vi "多帧接收机制(EV05).vi"(0 "can卡类型":u8, 1 "设备索引号":u8, 2 "CAN端口":u8, 3 "VCI_Receive":T1 {"Rsv3" max=0 format="%x"; "Rsv2" min=101 format="%x"; "Rsv1" format="%x"; "Data8" format="%x"; "Data7" format="%x"; "Data6" format="%x"; "Data5" format="%x"; "Data4" format="%x"; "Data3" format="%x"; "Data2" format="%x"; "Data1" format="%x"; "DataLen" format="%x"; "ExternFlag" format="%x"; "RemoteFlag" format="%x"; "SendType" format="%x"; "TimeFlag" format="%x"; "TimeStamp" format="%x"; "ID" format="%x"}, 4 "命令":u32 format="%x", 5 "板号":u32 format="%x", 7 "写?":bool, 9 "命令序号":u8) -> (13 "错误信号":bool, 14 "错误代码":i32, 15 "多帧数据长度":i32, 16 "命令序号":u8, 17 "输出数组":u8[](array[numeric]), 18 "读错误代码":u8[](array[numeric]), 19 "结束信号":bool)   [LabVIEW 2013]
panel:
  in  "最大帧号":i32
  out "多帧个数":i32
  out "长度1":i32
  out "接收完成":bool
  in  "多帧计时":bool
  in  "Reset 2":bool caption="重置"
  in  "Reset":bool caption="重置"
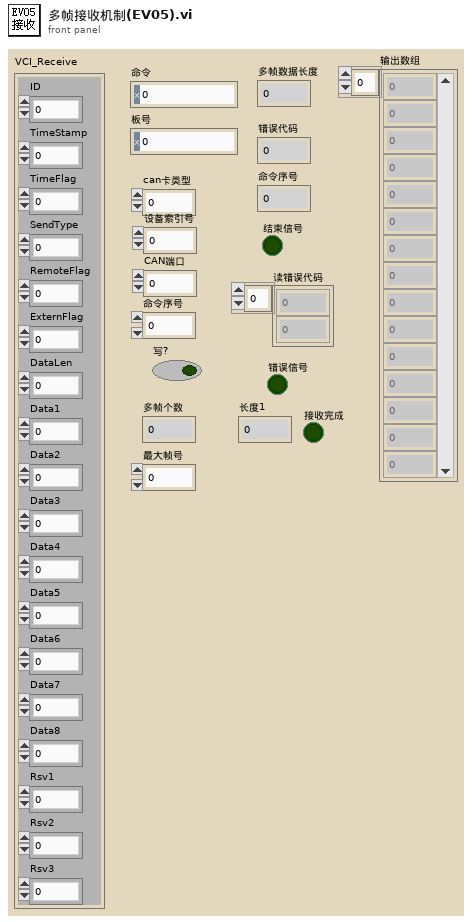
[diagram p1: front panel]
types:
  T1 = cluster{"ID":u32, "TimeStamp":u32, "TimeFlag":u8, "SendType":u8, "RemoteFlag":u8, "ExternFlag":u8, "DataLen":u8, "Data1":u8, "Data2":u8, "Data3":u8, "Data4":u8, "Data5":u8, "Data6":u8, "Data7":u8, "Data8":u8, "Rsv1":u8, "Rsv2":u8, "Rsv3":u8}
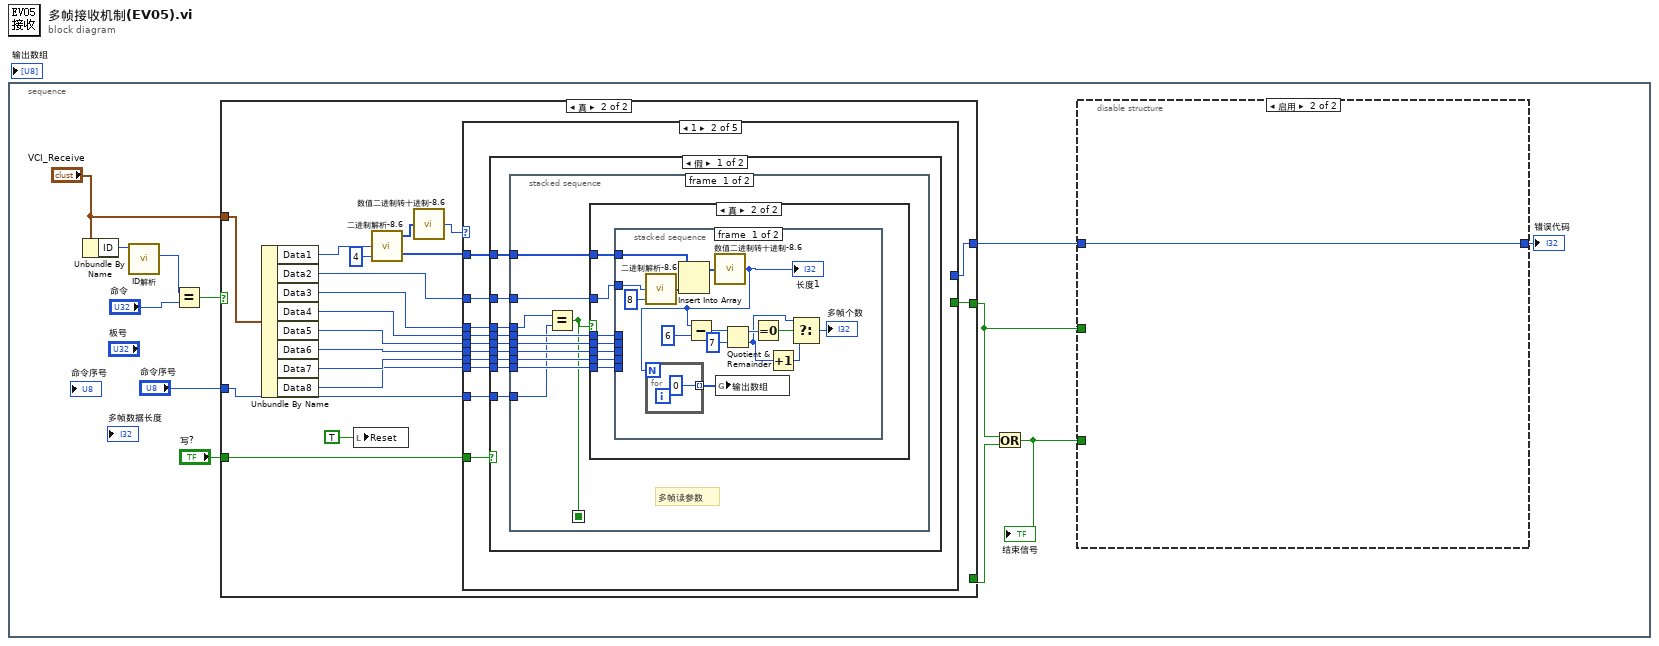
[diagram p0: block diagram]
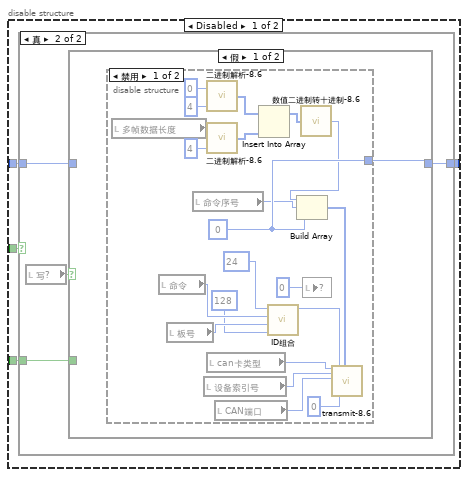
[diagram p2: hidden frame]
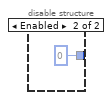
[diagram p4: hidden frame]
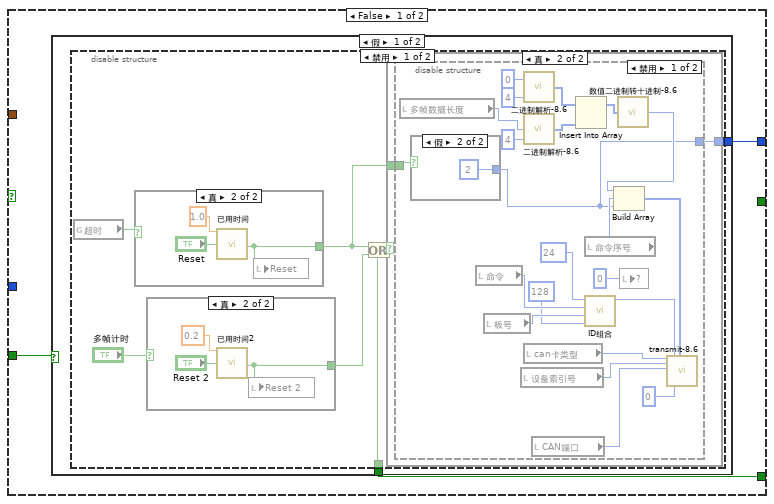
[diagram p6: hidden frame]
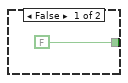
[diagram p8: hidden frame]
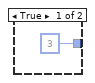
[diagram p10: hidden frame]
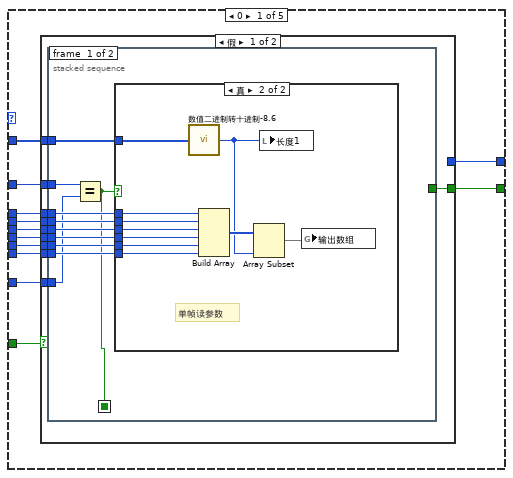
[diagram p14: hidden frame]
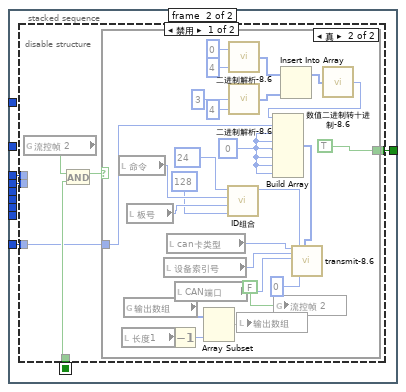
[diagram p16: hidden frame]
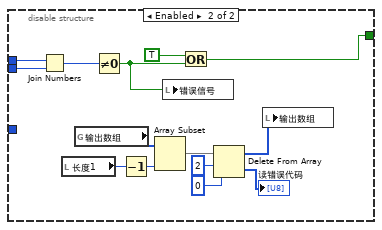
[diagram p18: hidden frame]
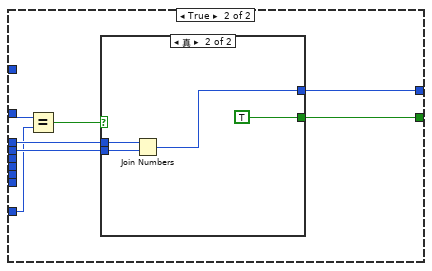
[diagram p19: hidden frame]
diagram:
  n1 = stacked-sequence {
    frame #0 {
      n2 = Unbundle By Name("VCI_Receive") -> ("ID"=w12:u32)
      n3 = call "ID解析.vi"("ID"=w12) -> ("PF(2)"=w11:i32)  [unwired: 10 out]
      n4 = Equal?(x=w11, y="命令") -> (x = y?=w5:bool)
      n5 = case shown="真" w5 {
        tunnel: "VCI_Receive" -> [_ w108]
        tunnel: [_ w94] -> w8
        tunnel: [w49 _] -> w4
        tunnel: [w48 w93] -> w7
        tunnel: "写?" -> [w47 w92]
        tunnel: "命令序号" -> [_ w91]
        frame False {
          n6 = case shown="假" w47 {
            tunnel: [w51 _] -> w49
            tunnel: [w50 _] -> w48
            frame False {
              n7 = disable-structure shown="禁用" {
                disable-tunnel: [w54 _] -> w51
                disable-tunnel: [w53 _] -> w50
                frame Disabled {
                  n8 = global read "EV05全局变量1.vi" "超时"() -> (w52:bool)
                  n9 = case shown="真" w52 {
                    tunnel: [_ w60] -> w56
                    frame False {
                    }
                    frame True {
                      n10 = call "已用时间"("Time Target (s)"=1.0, "Reset"="Reset") -> ("Time has Elapsed"=w60:bool)  [unwired: 3 in, 14 out]
                      n11 = local write "Reset"(w60) -> ()
                    }
                  }
                  n12 = case shown="真" "多帧计时" {
                    tunnel: [FALSE ("Time has Elapsed") w62] -> w55
                    frame False {
                    }
                    frame True {
                      n13 = call "已用时间2"("Time Target (s)"=0.2, "Reset"="Reset 2") -> ("Time has Elapsed"=w62:bool)  [unwired: 3 in, 14 out]
                      n14 = local write "Reset 2"(w62) -> ()
                    }
                  }
                  n15 = Or(x=w56, y=w55) -> (x .or. y?=w54:bool)
                  n16 = case shown="真" w54 {
                    tunnel: w56 -> [_ w66]
                    tunnel: [_ w65] -> w53
                    frame False {
                    }
                    frame True {
                      n17 = disable-structure shown="禁用" {
                        disable-tunnel: w66 -> [w81 _]
                        disable-tunnel: [w70 _] -> w65
                        frame Disabled {
                          n18 = local read "多帧数据长度"() -> (w72:i32)
                          n19 = case shown="假" w81 {
                            tunnel: [3 ("元素") 2 ("元素")] -> w70
                            frame True {
                            }
                            frame False {
                            }
                          }
                          n20 = local read "命令"() -> (w84:u32)
                          n21 = local read "板号"() -> (w69:u32)
                          n22 = local read "设备索引号"() -> (w87:u8)
                          n23 = call "二进制解析-8.6.vi"("索引"=4, "数值"=0) -> ("低位子数组"=w75:i32[])  [unwired: 3 out]
                          n24 = call "二进制解析-8.6.vi"("索引"=4, "数值"=w72) -> ("低位子数组"=w74:i32[])  [unwired: 3 out]
                          n25 = local read "can卡类型"() -> (w88:u8)
                          n26 = local read "CAN端口"() -> (w86:u8)
                          n27 = Insert Into Array(array=w75, new element=w74) -> (w73:i32[])  [unwired: 1 in]
                          n28 = local read "命令序号"() -> (w80:u8)
                          n29 = call "ID组合.vi"("SA(4)"=128 ("PDU(1)"), "PS(3)"=w69, "PF(2)"=w84, "PDU(1)"=24) -> ("ID"=w83:i32)  [unwired: 7 out]
                          n30 = call "数值二进制转十进制-8.6.vi"("子数组"=w73) -> ("十进制数值"=w71:i32)  [unwired: 4 out]
                          n31 = Build Array(w71, w80, w70) -> (w82:i32[])
                          n32 = local write item#-1(u8 0 ("计数")) -> ()
                          n33 = call "transmit-8.6.vi"("can卡类型"=w88, "设备索引号"=w87, "CAN端口"=w86, "ID"=w83, "SendType"=u8 0, "Data"=w82) -> ()  [unwired: 3 in, 11 out]
                        }
                        frame Enabled {
                        }
                      }
                    }
                  }
                }
                frame Enabled {
                }
              }
            }
            frame True {
            }
          }
        }
        frame True {
          n34 = Unbundle By Name(w108) -> ("Data1"=w107:u8, "Data2"=w103:u8, "Data3"=w101:u8, "Data4"=w100:u8, "Data5"=w99:u8, "Data6"=w98:u8, "Data7"=w97:u8, "Data8"=w96:u8)
          n35 = local write "Reset"(TRUE ("Reset")) -> ()
          n36 = call "二进制解析-8.6.vi"("索引"=4, "数值"=w107) -> ("低位子数组"=w102:i32[], "高位子数组"=w105:i32[])  [unwired: 2 out]
          n37 = call "数值二进制转十进制-8.6.vi"("子数组"=w105) -> ("十进制数值"=w104:i32)  [unwired: 4 out]
          n38 = case shown="1" w104 {
            tunnel: w103 -> [w120 w221 w307 _ _]
            tunnel: w102 -> [w119 w220 w309 _ _]
            tunnel: w101 -> [w113 w219 w308 _ _]
            tunnel: w100 -> [w118 w218 w306 _ _]
            tunnel: w99 -> [w117 w217 w305 _ _]
            tunnel: w98 -> [w116 w216 w304 _ _]
            tunnel: w97 -> [w115 w215 w303 _ _]
            tunnel: w96 -> [w114 w214 w302 _ _]
            tunnel: [w110 _ w299 _ _] -> w94
            tunnel: [w112 _ _ _ _] -> w93
            tunnel: w92 -> [w111 w213 w298 _ _]
            tunnel: w91 -> [w109 w212 _ _ _]
            frame 0 {
              n39 = case shown="假" w111 {
                tunnel: w120 -> [w130 w203]
                tunnel: w119 -> [w129 _]
                tunnel: w118 -> [w128 w205]
                tunnel: w117 -> [w127 _]
                tunnel: w116 -> [w126 _]
                tunnel: w115 -> [w125 _]
                tunnel: w114 -> [w124 _]
                tunnel: w113 -> [w123 w206]
                tunnel: [_ w207] -> w112
                tunnel: [w122 w204] -> w110
                tunnel: w109 -> [w121 w202]
                frame False {
                  n40 = stacked-sequence {
                    seq-local: [w131 _] -> [_ w154]
                    tunnel: w130 -> [w133 _]
                    tunnel: w129 -> [w140 _]
                    tunnel: w128 -> [w139 w151]
                    tunnel: w127 -> [w138 _]
                    tunnel: w126 -> [w137 _]
                    tunnel: w125 -> [w136 _]
                    tunnel: w124 -> [w135 _]
                    tunnel: w123 -> [w134 w152]
                    tunnel: [_ w155] -> w122
                    tunnel: w121 -> [w132 w153]
                    frame #0 {
                      n41 = Equal?(x=w133, y=w132) -> (x = y?=w131:bool)
                      n42 = case shown="真" w131 {
                        tunnel: w140 -> [_ w150]
                        tunnel: w139 -> [_ w149]
                        tunnel: w138 -> [_ w148]
                        tunnel: w137 -> [_ w147]
                        tunnel: w136 -> [_ w146]
                        tunnel: w135 -> [_ w145]
                        tunnel: w134 -> [_ w144]
                        frame False {
                        }
                        frame True {
                          # "单帧读参数"
                          n43 = call "数值二进制转十进制-8.6.vi"("子数组"=w150) -> ("十进制数值"=w142:i32)  [unwired: 4 out]
                          n44 = Build Array(w144, w149, w148, w147, w146, w145) -> (w143:u8[])
                          n45 = Array Subset(array=w143, length=w142) -> (w141:u8[])  [unwired: 1 in]
                          n46 = local write "长度1"(w142) -> ()
                          n47 = global write "EV05全局变量1.vi" "输出数组"(w141) -> ()
                        }
                      }
                    }
                    frame #1 {
                      n48 = disable-structure shown="禁用" {
                        disable-tunnel: [w160 w189] -> w155
                        disable-tunnel: w154 -> [w159 _]
                        disable-tunnel: w153 -> [w156 _]
                        disable-tunnel: w152 -> [_ w195]
                        disable-tunnel: w151 -> [_ w196]
                        frame Disabled {
                          n49 = global read "EV05全局变量1.vi" "流控帧 2"() -> (w157:bool)
                          n50 = And(x=w157, y=w159) -> (x .and. y?=w158:bool)
                          n51 = case shown="真" w158 {
                            tunnel: [_ TRUE] -> w160
                            tunnel: w156 -> [_ w163]
                            frame False {
                            }
                            frame True {
                              w179 = 0 ("元素")
                              n52 = local read "命令"() -> (w182:u32)
                              n53 = local read "长度1"() -> (w165:i32)
                              n54 = global read "EV05全局变量1.vi" "输出数组"() -> (w167:u8[])
                              n55 = local read "板号"() -> (w171:u32)
                              n56 = local read "设备索引号"() -> (w185:u8)
                              n57 = local read "can卡类型"() -> (w186:u8)
                              n58 = Decrement(x=w165) -> (x-1=w164:i32)
                              n59 = local read "CAN端口"() -> (w184:u8)
                              n60 = Array Subset(array=w167, length=w164) -> (w166:u8[])  [unwired: 1 in]
                              n61 = call "ID组合.vi"("SA(4)"=128 ("PDU(1)"), "PS(3)"=w171, "PF(2)"=w182, "PDU(1)"=24) -> ("ID"=w181:i32)  [unwired: 7 out]
                              n62 = call "二进制解析-8.6.vi"("索引"=4, "数值"=0) -> ("低位子数组"=w175:i32[])  [unwired: 3 out]
                              n63 = call "二进制解析-8.6.vi"("索引"=4, "数值"=3) -> ("低位子数组"=w172:i32[])  [unwired: 3 out]
                              n64 = local write "输出数组"(w166) -> ()
                              n65 = global write "EV05全局变量1.vi" "流控帧 2"(FALSE ("流控帧 2")) -> ()
                              n66 = Insert Into Array(array=w175, new element=w172) -> (w174:i32[])  [unwired: 1 in]
                              n67 = call "数值二进制转十进制-8.6.vi"("子数组"=w174) -> ("十进制数值"=w173:i32)  [unwired: 4 out]
                              n68 = Build Array(w173, w163, w179, w179, w179, w179, w179, w179) -> (w180:i32[])
                              n69 = call "transmit-8.6.vi"("can卡类型"=w186, "设备索引号"=w185, "CAN端口"=w184, "ID"=w181, "SendType"=u8 0, "Data"=w180) -> ()  [unwired: 3 in, 11 out]
                            }
                          }
                        }
                        frame Enabled {
                          n70 = Join Numbers(hi=w195, lo=w196) -> ((hi.lo)=w194:u16)
                          n71 = local read "长度1"() -> (w198:i32)
                          n72 = global read "EV05全局变量1.vi" "输出数组"() -> (w200:u8[])
                          n73 = Not Equal To 0?(x=w194) -> (x != 0?=w187:bool)
                          n74 = Decrement(x=w198) -> (x-1=w197:i32)
                          n75 = Array Subset(array=w200, length=w197) -> (w199:u8[])  [unwired: 1 in]
                          n76 = local write "错误信号"(w187) -> ()
                          n77 = Or(x=TRUE, y=w187) -> (x .or. y?=w189:bool)
                          n78 = Delete From Array(array=w199, length=2 ("长度"), index=0 ("索引")) -> (deleted portion=→"读错误代码":u8[], array with subset deleted=w193:u8[])
                          n79 = local write "输出数组"(w193) -> ()
                        }
                      }
                    }
                  }
                }
                frame True {
                  n80 = Equal?(x=w203, y=w202) -> (x = y?=w201:bool)
                  n81 = case shown="真" w201 {
                    tunnel: [_ w211] -> w207
                    tunnel: w206 -> [_ w210]
                    tunnel: w205 -> [_ w209]
                    tunnel: [_ TRUE] -> w204
                    frame False {
                    }
                    frame True {
                      n82 = Join Numbers(hi=w210, lo=w209) -> ((hi.lo)=w211:u16)
                    }
                  }
                }
              }
            }
            frame 1 {
              n83 = case shown="假" w213 {
                tunnel: w221 -> [w230 _]
                tunnel: w220 -> [w229 _]
                tunnel: w219 -> [w228 _]
                tunnel: w218 -> [w227 _]
                tunnel: w217 -> [w226 _]
                tunnel: w216 -> [w225 _]
                tunnel: w215 -> [w224 _]
                tunnel: w214 -> [w223 _]
                tunnel: w212 -> [w222 _]
                frame False {
                  n84 = stacked-sequence {
                    seq-local: [w231 _] -> [_ w276]
                    tunnel: w230 -> [w240 _]
                    tunnel: w229 -> [w239 _]
                    tunnel: w228 -> [w233 _]
                    tunnel: w227 -> [w238 _]
                    tunnel: w226 -> [w237 _]
                    tunnel: w225 -> [w236 _]
                    tunnel: w224 -> [w235 _]
                    tunnel: w223 -> [w234 _]
                    tunnel: w222 -> [w232 _]
                    frame #0 {
                      # "多帧读参数"
                      n85 = Equal?(x=w233, y=w232) -> (x = y?=w231:bool)
                      n86 = case shown="真" w231 {
                        tunnel: w240 -> [_ w247]
                        tunnel: w239 -> [_ w246]
                        tunnel: w238 -> [_ w245]
                        tunnel: w237 -> [_ w244]
                        tunnel: w236 -> [_ w243]
                        tunnel: w235 -> [_ w242]
                        tunnel: w234 -> [_ w241]
                        frame False {
                        }
                        frame True {
                          n87 = stacked-sequence {
                            tunnel: w247 -> [w261 _]
                            tunnel: w246 -> [w259 _]
                            tunnel: w245 -> [_ w273]
                            tunnel: w244 -> [_ w272]
                            tunnel: w243 -> [_ w271]
                            tunnel: w242 -> [_ w270]
                            tunnel: w241 -> [_ w269]
                            frame #0 {
                              n88 = call "二进制解析-8.6.vi"("索引"=8, "数值"=w261) -> ("低位子数组"=w260:i32[])  [unwired: 3 out]
                              n89 = Insert Into Array(array=w259, new element=w260) -> (w258:i32[])  [unwired: 1 in]
                              n90 = call "数值二进制转十进制-8.6.vi"("子数组"=w258) -> ("十进制数值"=w256:i32)  [unwired: 4 out]
                              "长度1" <- w256
                              n91 = for {
                                N: w256 -> [_]
                                tunnel: [u8 0] -> w257 mode=indexing
                              }
                              n92 = Subtract(x=w256, y=6) -> (x-y=w254:i32)
                              n93 = global write "EV05全局变量1.vi" "输出数组"(w257) -> ()
                              n94 = Quotient & Remainder(x=w254, y=7) -> (x-y*floor(x/y)=w252:i32, floor(x/y)=w250:i32)
                              n95 = Equal To 0?(x=w252) -> (x = 0?=w251:bool)
                              n96 = Increment(x=w250) -> (x+1=w249:i32)
                              n97 = Select(t=w250, s=w251, f=w249) -> (s? t:f=→"多帧个数":i32)
                            }
                            frame #1 {
                              # "收第一帧5字节数据"
                              n98 = Build Array(w273, w272, w271, w270, w269) -> (w267:u8[])
                              n99 = global read "EV05全局变量1.vi" "输出数组"() -> (w268:u8[])
                              n100 = local write "最大帧号"(1 ("最大帧号")) -> ()
                              n101 = Replace Array Subset(array=w268, new element=w267, index=0 ("索引")) -> (w266:u8[])
                              n102 = global write "EV05全局变量1.vi" "输出数组"(w266) -> ()
                            }
                          }
                        }
                      }
                    }
                    frame #1 {
                      n103 = global read "EV05全局变量1.vi" "流控帧 2"() -> (w274:bool)
                      n104 = And(x=w274, y=w276) -> (x .and. y?=w275:bool)
                      n105 = case shown="真" w275 {
                        frame False {
                        }
                        frame True {
                          w283 = 0 ("元素")
                          n106 = local read "命令"() -> (w284:u32)
                          n107 = local read "板号"() -> (w280:u32)
                          n108 = call "ID组合.vi"("SA(4)"=145 ("PDU(1)"), "PS(3)"=w280, "PF(2)"=w284, "PDU(1)"=24) -> ("ID"=w286:i32)  [unwired: 7 out]
                          n109 = call "二进制解析-8.6.vi"("索引"=4, "数值"=3) -> ("低位子数组"=w291:i32[])  [unwired: 3 out]
                          n110 = call "二进制解析-8.6.vi"("索引"=4, "数值"=0) -> ("低位子数组"=w290:i32[])  [unwired: 3 out]
                          n111 = Insert Into Array(array=w291, new element=w290) -> (w289:i32[])  [unwired: 1 in]
                          n112 = global write "EV05全局变量1.vi" "流控帧 2"(FALSE ("流控")) -> ()
                          n113 = call "数值二进制转十进制-8.6.vi"("子数组"=w289) -> ("十进制数值"=w288:i32)  [unwired: 4 out]
                          n114 = Build Array(w288, w283, 20 ("元素"), w283, w283, w283, w283, w283) -> (w287:i32[])
                          n115 = call "transmit-8.6.vi"("can卡类型"="can卡类型", "设备索引号"="设备索引号", "CAN端口"="CAN端口", "ID"=w286, "SendType"=u8 0, "Data"=w287) -> ()  [unwired: 3 in, 11 out]
                        }
                      }
                    }
                  }
                }
                frame True {
                }
              }
            }
            frame 2 {
              n116 = case shown="假" w298 {
                tunnel: w309 -> [w318 _]
                tunnel: w308 -> [w317 _]
                tunnel: w307 -> [w316 _]
                tunnel: w306 -> [w315 _]
                tunnel: w305 -> [w314 _]
                tunnel: w304 -> [w313 _]
                tunnel: w303 -> [w312 _]
                tunnel: w302 -> [w311 _]
                tunnel: [w310 _] -> w299
                frame False {
                  n117 = stacked-sequence {
                    seq-local: [w320 _] -> [_ w338]
                    seq-local: [w319 _] -> [_ w340]
                    tunnel: w318 -> [w337 _]
                    tunnel: w317 -> [w336 _]
                    tunnel: w316 -> [w335 _]
                    tunnel: w315 -> [w334 _]
                    tunnel: w314 -> [w333 _]
                    tunnel: w313 -> [w332 _]
                    tunnel: w312 -> [w331 _]
                    tunnel: w311 -> [w330 _]
                    tunnel: [_ w354] -> w310
                    frame #0 {
                      n118 = call "数值二进制转十进制-8.6.vi"("子数组"=w337) -> ("十进制数值"=w322:i32)  [unwired: 4 out]
                      n119 = Build Array(w335, w336, w334, w333, w332, w331, w330) -> (w323:u8[])
                      n120 = Decrement(x=w322) -> (x-1=w327:i32)
                      n121 = Multiply(x=w327, y=7) -> (x*y=w326:i32)
                      n122 = Max & Min(x="最大帧号", y=w322) -> (max(x,y)=w320:i32)  [unwired: 1 out]
                      n123 = Add(x=w326, y=5) -> (x+y=w324:i32)
                      n124 = global read "EV05全局变量1.vi" "输出数组"() -> (w329:u8[])
                      n125 = Replace Array Subset(array=w329, new element=w323, index=w324) -> (w319:u8[])
                      n126 = local write "最大帧号"(w320) -> ()
                      n127 = global write "EV05全局变量1.vi" "输出数组"(w319) -> ()
                    }
                    frame #1 {
                      n128 = local read "长度1"() -> (w352:i32)
                      n129 = local read "多帧个数"() -> (w339:i32)
                      n130 = Decrement(x=w352) -> (x-1=w351:i32)
                      n131 = Array Subset(array=w340, length=w351) -> (w353:u8[])  [unwired: 1 in]
                      n132 = Equal?(x=w338, y=w339) -> (x = y?=w355:bool)
                      "接收完成" <- w355
                      n133 = Delete From Array(array=w353, length=2 ("长度"), index=0 ("索引")) -> (deleted portion=w347:u8[], array with subset deleted=w350:u8[])
                      n134 = local write "读错误代码"(w347) -> ()
                      n135 = Index Array(array=w347, index #1=0 ("索引"), index #2=1 ("索引")) -> (element #1=w343:u8, element #2=w344:u8)
                      n136 = local write "输出数组"(w350) -> ()
                      n137 = Join Numbers(hi=w343, lo=w344) -> ((hi.lo)=w342:u16)
                      n138 = Not Equal To 0?(x=w342) -> (x != 0?=w341:bool)
                      "错误信号" <- w341
                      n139 = Or(x=w355, y=w341) -> (x .or. y?=w354:bool)
                    }
                  }
                }
                frame True {
                }
              }
              n140 = local write "多帧计时"(TRUE ("多帧计时")) -> ()
              n141 = local write "Reset 2"(TRUE ("Reset 2")) -> ()
            }
            frame 3 {
              n142 = global write "EV05全局变量1.vi" "流控帧"(TRUE ("Reset")) -> ()
            }
            frame 4, Default {
            }
          }
        }
      }
      n143 = Or(x=w8, y=w4) -> (x .or. y?=w2:bool)
      "结束信号" <- w2
      n144 = disable-structure shown="启用" {
        disable-tunnel: w8 -> [w16 _]
        disable-tunnel: w7 -> [w15 w46]
        disable-tunnel: [w14 w46] -> w6
        disable-tunnel: w2 -> [w13 _]
        frame Disabled {
          n145 = case shown="真" w16 {
            tunnel: w15 -> [w17 w19]
            tunnel: [w17 w21] -> w14
            tunnel: w13 -> [_ w18]
            frame False {
            }
            frame True {
              n146 = local read "写?"() -> (w20:bool)
              n147 = case shown="假" w20 {
                tunnel: [w22 w45] -> w21
                tunnel: w19 -> [_ w45]
                tunnel: w18 -> [_ _]
                frame False {
                  n148 = disable-structure shown="禁用" {
                    disable-tunnel: [w43 0 ("元素")] -> w22
                    frame Disabled {
                      w43 = 0 ("元素")
                      n149 = local read "多帧数据长度"() -> (w41:i32)
                      n150 = local read "命令"() -> (w30:u32)
                      n151 = local read "板号"() -> (w25:u32)
                      n152 = local read "命令序号"() -> (w33:u8)
                      n153 = local read "设备索引号"() -> (w27:u8)
                      n154 = call "二进制解析-8.6.vi"("索引"=4, "数值"=0) -> ("低位子数组"=w38:i32[])  [unwired: 3 out]
                      n155 = call "二进制解析-8.6.vi"("索引"=4, "数值"=w41) -> ("低位子数组"=w39:i32[])  [unwired: 3 out]
                      n156 = local read "can卡类型"() -> (w26:u8)
                      n157 = local read "CAN端口"() -> (w28:u8)
                      n158 = Insert Into Array(array=w38, new element=w39) -> (w40:i32[])  [unwired: 1 in]
                      n159 = call "ID组合.vi"("SA(4)"=128 ("PDU(1)"), "PS(3)"=w25, "PF(2)"=w30, "PDU(1)"=24) -> ("ID"=w31:i32)  [unwired: 7 out]
                      n160 = call "数值二进制转十进制-8.6.vi"("子数组"=w40) -> ("十进制数值"=w42:i32)  [unwired: 4 out]
                      n161 = Build Array(w42, w33, w43) -> (w32:i32[])
                      n162 = local write item#-1(u8 0 ("计数")) -> ()
                      n163 = call "transmit-8.6.vi"("can卡类型"=w26, "设备索引号"=w27, "CAN端口"=w28, "ID"=w31, "SendType"=u8 0, "Data"=w32) -> ()  [unwired: 3 in, 11 out]
                    }
                    frame Enabled {
                    }
                  }
                }
                frame True {
                }
              }
            }
          }
        }
        frame Enabled {
        }
      }
      "错误代码" <- w6
    }
  }
